vi "Format System.vi"   [LabVIEW 2020, in "nisyscfg.lvlib"]
doc: "Erases all data from the primary hard drive of a system."
uses:
  <vilib>/nisyscfg/nisyscfg.lvlib
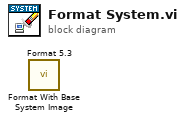
[diagram p0: block diagram]
diagram:
  n1 = call <vilib>:"Format With Base System Image.vi"() -> ()  [unwired: 10 in, 2 out]
  n2 = call <vilib>:"Format 5.3.vi"() -> ()  [unwired: 10 in, 2 out]
